vi "modbus_crc.vi"(1 "字符串":string="shuju1") -> (0 "十六进制整型字符串":string)   [LabVIEW 2023]
panel:
  out "数值":i32 format="%x"
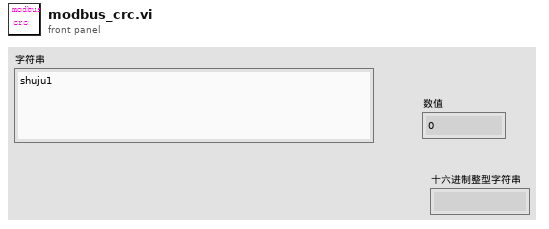
[diagram p1: front panel]
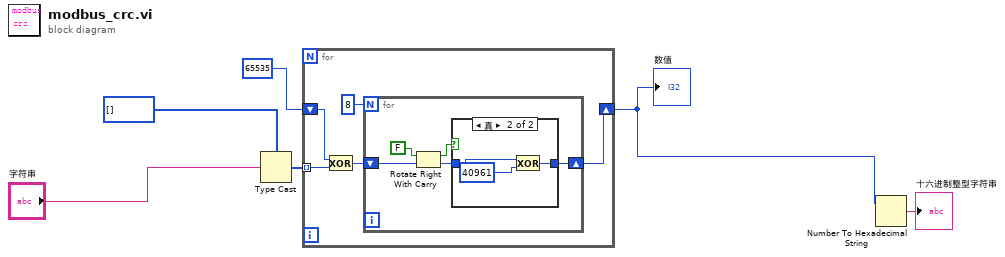
[diagram p0: block diagram]
diagram:
  n1 = Type Cast(type=u8[] [], x="字符串") -> (*(type *) &x=w6:u8[])
  n2 = for {
    tunnel: w6 -> [w7] mode=indexing
    shift-right: [w9] -> w1
    shift-left: u16 65535 -> [w11]
    n3 = Exclusive Or(1:w7, 2:w11) -> (0:w10:u16)
    n4 = for {
      N: 8 -> [_]
      shift-right: [w12] -> w9
      shift-left: w10 -> [w16]
      n5 = Rotate Right With Carry(2:w16, 3:FALSE ("进位")) -> (0:w13:u16, 1:w14:bool)
      n6 = case shown="真" w14 {
        tunnel: w13 -> [w17 w20]
        tunnel: [w17 w18] -> w12
        frame False {
        }
        frame True {
          n7 = Exclusive Or(1:u16 40961 ("y"), 2:w20) -> (0:w18:u16)
        }
      }
    }
  }
  "数值" <- w1
  n8 = Number To Hexadecimal String(2:w1) -> (0:→"十六进制整型字符串":string)  [unwired: 1 in]
